vi "Measure_Single_Point_With_Compliance.vi"(8 "error in":errorcluster, 10 "Pin":string, 11 "niDMM in":refnum<class "niDMM.lvclass">) -> (0 "error out":errorcluster, 2 "DMM_Measurement_Results":T1, 3 "niDMM out":refnum<class "niDMM.lvclass">)   [LabVIEW 2020, in "niDMM.lvclass"]
uses:
  niDMM.lvclass
  DMM_Base/Typedef/DMM_Measurement_Results.ctl
  <vilib>/MeasurementLink/MeasurementLink niDMM/MeasurementLink niDMM.lvlib
  DMM_Base/DMM_Base.lvclass
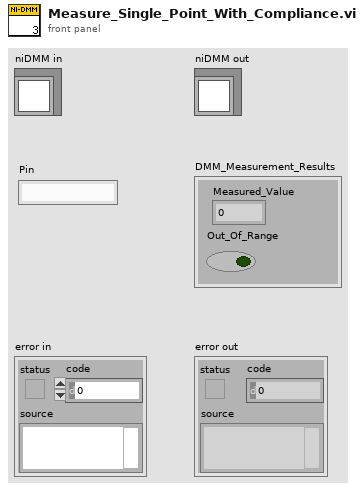
[diagram p1: front panel]
types:
  T1 = typedef "DMM_Base.lvclass/DMM_Measurement_Results.ctl" = cluster{"Measured_Value":dbl, "Out_Of_Range":bool}
  T2 = typedef "MeasurementLink niDMM.lvlib/Connection with Session.ctl" = cluster{"connection":T3, "session":refnum<k15>}
  T3 = typedef "MeasurementLink Session Management V1.lvlib/Session Reservation.lvclass/Connection.ctl" = cluster{"pin or relay name":string, "site":i32, "instrument type id":string, "channel":string}
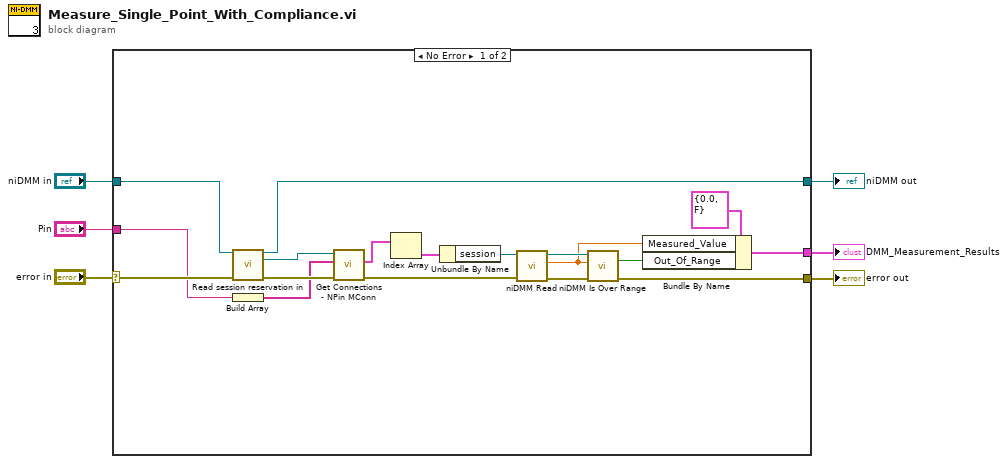
[diagram p0: block diagram]
diagram:
  n1 = case shown="No Error" "error in" {
    selector: "error in" -> [w16 w26]
    tunnel: [w15 w26] -> w5
    tunnel: "niDMM in" -> [w14 w25]
    tunnel: [w13 w25] -> w3
    tunnel: [w9 _] -> w2
    tunnel: "Pin" -> [w8 _]
    frame No Error {
      n2 = call-dynamic "Read session reservation in.vi"("AbstractDMM in"=w14, "error in (no error)"=w16) -> ("AbstractDMM out"=w13:refnum<class "niDMM.lvclass">, "MeasurementLink Session Management V1.lvlib:Session Reservation.lvclass"=w19:refnum<class "Session Reservation.lvclass">, "error out"=w20:errorcluster)  [unwired: 11 in]
      n3 = Build Array(w8) -> (w7:string[])
      n4 = call <vilib>:"Get Connections - NPin MConn.vi"("error in"=w20, "pin or relay names"=w7, "session reservation in"=w19) -> ("error out"=w21:errorcluster, "connections"=w22:T2[])  [unwired: 6 in, 1 out]
      n5 = Index Array(array=w22) -> (element=w23:T2)  [unwired: 1 in]
      n6 = Unbundle By Name(w23) -> ("session"=w24:refnum<k15>)
      n7 = call <instrlib>:"niDMM Read.vi"("error in (no error)"=w21, "instrument handle"=w24) -> ("error out"=w17:errorcluster, "Measurement"=w10:dbl, "instrument handle out"=w18:refnum<k15>)  [unwired: 7 in]
      n8 = call <instrlib>:"niDMM Is Over Range.vi"("error in (no error)"=w17, "Measurement"=w10, "instrument handle"=w18) -> ("error out"=w15:errorcluster, "Over Range?"=w11:bool)  [unwired: 6 in, 1 out]
      n9 = Bundle By Name(cluster=T1 {"Measured_Value"=0.0, "Out_Of_Range"=FALSE} ("DMM_Measurement_Results"), "Measured_Value"=w10, "Out_Of_Range"=w11) -> (w9:T1)
    }
    frame Error {
    }
  }
  "error out" <- w5
  "niDMM out" <- w3
  "DMM_Measurement_Results" <- w2
